vi "信号定位2.vi"() -> ()   [LabVIEW 2013]
panel:
  in  "范围":dbl
  in  "速度m/s":dbl=1.0
  out "y":dbl
  out "x":dbl
  in  "y3":dbl
  in  "x3":dbl
  in  "y2":dbl
  in  "x2":dbl
  in  "y1":dbl
  in  "x1":dbl
  in  "signal 3":dbl
  in  "signal 2":dbl
  in  "signal 1":dbl
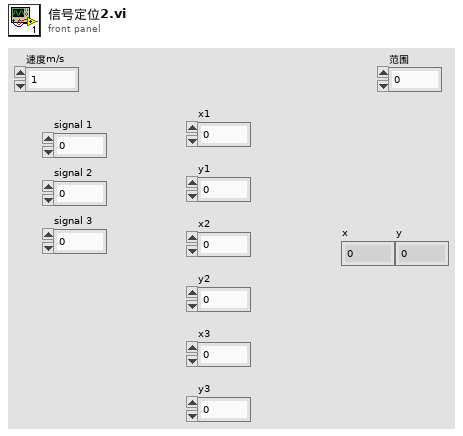
[diagram p1: front panel]
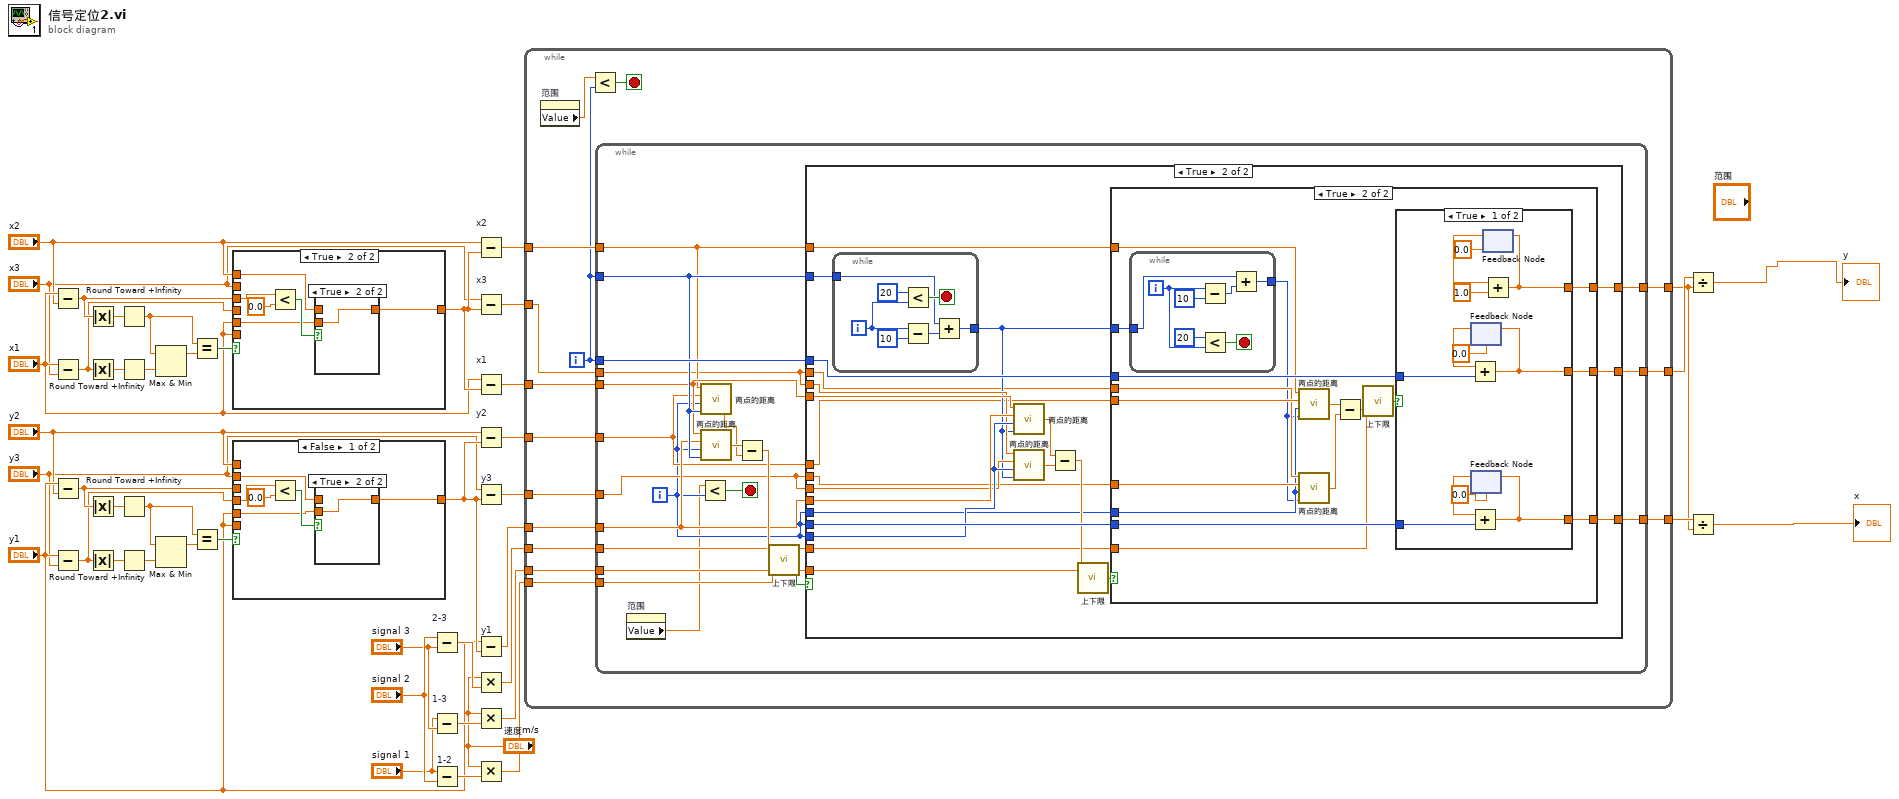
[diagram p0: block diagram]
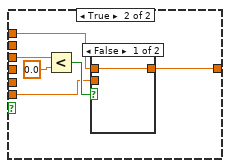
[diagram p3: hidden frame]
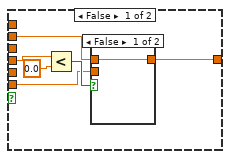
[diagram p5: hidden frame]
diagram:
  n1 = Subtract(x="x1", y="x2") -> (x-y=w24:dbl)
  n2 = Subtract(x="x1", y="x3") -> (x-y=w23:dbl)
  n3 = Subtract(x="y1", y="y2") -> (x-y=w26:dbl)
  n4 = Subtract(x="y1", y="y3") -> (x-y=w25:dbl)
  n5 = Absolute Value(x=w24) -> (abs(x)=w36:dbl)
  n6 = Absolute Value(x=w23) -> (abs(x)=w35:dbl)
  n7 = Absolute Value(x=w26) -> (abs(x)=w28:dbl)
  n8 = Absolute Value(x=w25) -> (abs(x)=w27:dbl)
  n9 = Round Toward +Infinity(x=w36) -> (ceil(x): smallest int >= x=w32:dbl)
  n10 = Round Toward +Infinity(x=w35) -> (ceil(x): smallest int >= x=w42:dbl)
  n11 = Round Toward +Infinity(x=w28) -> (ceil(x): smallest int >= x=w29:dbl)
  n12 = Round Toward +Infinity(x=w27) -> (ceil(x): smallest int >= x=w41:dbl)
  n13 = Max & Min(x=w32, y=w42) -> (max(x,y)=w33:dbl)  [unwired: 1 out]
  n14 = Max & Min(x=w29, y=w41) -> (max(x,y)=w30:dbl)  [unwired: 1 out]
  n15 = Equal?(x=w32, y=w33) -> (x = y?=w34:bool)
  n16 = Equal?(x=w29, y=w30) -> (x = y?=w31:bool)
  n17 = case shown="True" w34 {
    tunnel: w24 -> [_ w57]
    tunnel: "x1" -> [_ w56]
    tunnel: [w47 w55] -> w22
    tunnel: "x2" -> [_ w54]
    tunnel: w23 -> [w49 _]
    tunnel: "x1" -> [w48 _]
    tunnel: "x3" -> [w46 _]
    frame False {
      n18 = Less?(x=w49, y=0.0) -> (x < y?=w50:bool)
      n19 = case shown="False" w50 {
        tunnel: w48 -> [_ w53]
        tunnel: [w52 w53] -> w47
        tunnel: w46 -> [w52 _]
        frame False {
        }
        frame True {
        }
      }
    }
    frame True {
      n20 = Less?(x=w57, y=0.0) -> (x < y?=w59:bool)
      n21 = case shown="True" w59 {
        tunnel: w56 -> [_ w61]
        tunnel: [w60 w61] -> w55
        tunnel: w54 -> [w60 _]
        frame False {
        }
        frame True {
        }
      }
    }
  }
  n22 = case shown="False" w31 {
    tunnel: w26 -> [_ w73]
    tunnel: "y1" -> [_ w72]
    tunnel: [w63 w71] -> w18
    tunnel: "y2" -> [_ w70]
    tunnel: w25 -> [w65 _]
    tunnel: "y1" -> [w64 _]
    tunnel: "y3" -> [w62 _]
    frame False {
      n23 = Less?(x=w65, y=0.0) -> (x < y?=w66:bool)
      n24 = case shown="True" w66 {
        tunnel: w64 -> [_ w69]
        tunnel: [w68 w69] -> w63
        tunnel: w62 -> [w68 _]
        frame False {
        }
        frame True {
        }
      }
    }
    frame True {
      n25 = Less?(x=w73, y=0.0) -> (x < y?=w75:bool)
      n26 = case shown="False" w75 {
        tunnel: w72 -> [_ w77]
        tunnel: [w76 w77] -> w71
        tunnel: w70 -> [w76 _]
        frame False {
        }
        frame True {
        }
      }
    }
  }
  n27 = Subtract "2-3"(x="signal 2", y="signal 3") -> (x-y=w38:dbl)
  n28 = Subtract "1-3"(x="signal 1", y="signal 3") -> (x-y=w39:dbl)
  n29 = Subtract "1-2"(x="signal 1", y="signal 2") -> (x-y=w40:dbl)
  n30 = Subtract "x2"(x="x2", y=w22) -> (x-y=w12:dbl)
  n31 = Subtract "x3"(x="x3", y=w22) -> (x-y=w10:dbl)
  n32 = Subtract "x1"(x="x1", y=w22) -> (x-y=w14:dbl)
  n33 = Subtract "y2"(x="y2", y=w18) -> (x-y=w11:dbl)
  n34 = Subtract "y3"(x="y3", y=w18) -> (x-y=w9:dbl)
  n35 = Subtract "y1"(x="y1", y=w18) -> (x-y=w13:dbl)
  n36 = Multiply(x="速度m/s", y=w38) -> (x*y=w6:dbl)
  n37 = Multiply(x="速度m/s", y=w39) -> (x*y=w7:dbl)
  n38 = Multiply(x="速度m/s", y=w40) -> (x*y=w8:dbl)
  n39 = while {
    tunnel: w14 -> [w91]
    tunnel: w13 -> [w90]
    tunnel: w12 -> [w89]
    tunnel: w11 -> [w88]
    tunnel: w10 -> [w87]
    tunnel: w9 -> [w86]
    tunnel: w8 -> [w85]
    tunnel: w7 -> [w84]
    tunnel: w6 -> [w83]
    tunnel: [w81] -> w5
    tunnel: [w80] -> w4
    tunnel: [w79] -> w3
    i -> [w82]
    stop <- w92 stop-if-true
    n40 = property on="范围" class="DigNum (strict)"() -> ("Value"=w78:dbl)  [unwired: 2 in, 2 out]
    n41 = Less?(x=w78, y=w82) -> (x < y?=w92:bool)
    n42 = while {
      tunnel: w82 -> [w105]
      tunnel: w91 -> [w104]
      tunnel: w90 -> [w103]
      tunnel: w89 -> [w101]
      tunnel: w88 -> [w100]
      tunnel: w87 -> [w99]
      tunnel: w86 -> [w98]
      tunnel: w85 -> [w112]
      tunnel: w84 -> [w102]
      tunnel: w83 -> [w96]
      tunnel: w82 -> [w111]
      tunnel: [w110] -> w81
      tunnel: [w109] -> w80
      tunnel: [w108] -> w79
      i -> [w97]
      stop <- w113 stop-if-true
      n43 = property on="范围" class="DigNum (strict)"() -> ("Value"=w93:dbl)  [unwired: 2 in, 2 out]
      n44 = Less?(x=w93, y=w97) -> (x < y?=w113:bool)
      n45 = call "两点的距离.vi"("y2"=w105, "x2"=w97, "y1"=w100, "x1"=w101) -> ("de"=w94:dbl)
      n46 = call "两点的距离.vi"("y2"=w105, "x2"=w97, "y1"=w103, "x1"=w104) -> ("de"=w95:dbl)
      n47 = Subtract(x=w95, y=w94) -> (x-y=w106:dbl)
      n48 = call "上下限.vi"("要比较的"=w106, "范围的中心"=w112) -> ("T/F"=w107:bool)
      n49 = case shown="True" w107 {
        tunnel: w97 -> [_ w136]
        tunnel: w111 -> [_ w135]
        tunnel: [_ w134] -> w110
        tunnel: [_ w133] -> w109
        tunnel: [_ w132] -> w108
        tunnel: w105 -> [_ w131]
        tunnel: w97 -> [_ w130]
        tunnel: w104 -> [_ w129]
        tunnel: w103 -> [_ w128]
        tunnel: w99 -> [_ w127]
        tunnel: w98 -> [_ w126]
        tunnel: w102 -> [_ w124]
        tunnel: w101 -> [_ w121]
        tunnel: w100 -> [_ w120]
        tunnel: w99 -> [_ w119]
        tunnel: w98 -> [_ w118]
        tunnel: w97 -> [_ w117]
        tunnel: w96 -> [_ w116]
        frame False {
        }
        frame True {
          n50 = while {
            tunnel: w131 -> [w138]
            tunnel: [w137] -> w122
            i -> [w142]
            stop <- w141 stop-if-true
            n51 = Less?(x=20, y=w142) -> (x < y?=w141:bool)
            n52 = Subtract(x=w142, y=10) -> (x-y=w139:i32)
            n53 = Add(x=w138, y=w139) -> (x+y=w137:i32)
          }
          n54 = call "两点的距离.vi"("y2"=w122, "x2"=w130, "y1"=w128, "x1"=w129) -> ("de"=w115:dbl)
          n55 = call "两点的距离.vi"("y2"=w122, "x2"=w130, "y1"=w126, "x1"=w127) -> ("de"=w114:dbl)
          n56 = Subtract(x=w115, y=w114) -> (x-y=w125:dbl)
          n57 = call "上下限.vi"("要比较的"=w125, "范围的中心"=w124) -> ("T/F"=w123:bool)
          n58 = case shown="True" w123 {
            tunnel: w136 -> [_ w160]
            tunnel: w135 -> [_ w159]
            tunnel: [_ w158] -> w134
            tunnel: [_ w157] -> w133
            tunnel: [_ w156] -> w132
            tunnel: w122 -> [_ w155]
            tunnel: w121 -> [_ w153]
            tunnel: w120 -> [_ w152]
            tunnel: w119 -> [_ w151]
            tunnel: w118 -> [_ w150]
            tunnel: w117 -> [_ w149]
            tunnel: w116 -> [_ w147]
            frame False {
            }
            frame True {
              n59 = while {
                tunnel: [w162] -> w148
                tunnel: w155 -> [w161]
                i -> [w166]
                stop <- w165 stop-if-true
                n60 = Subtract(x=w166, y=10) -> (x-y=w163:i32)
                n61 = Less?(x=20, y=w166) -> (x < y?=w165:bool)
                n62 = Add(x=w161, y=w163) -> (x+y=w162:i32)
              }
              n63 = call "两点的距离.vi"("y2"=w148, "x2"=w149, "y1"=w152, "x1"=w153) -> ("de"=w145:dbl)
              n64 = call "两点的距离.vi"("y2"=w148, "x2"=w149, "y1"=w150, "x1"=w151) -> ("de"=w144:dbl)
              n65 = Subtract(x=w145, y=w144) -> (x-y=w154:dbl)
              n66 = call "上下限.vi"("要比较的"=w154, "范围的中心"=w147) -> ("T/F"=w146:bool)
              n67 = case shown="True" w146 {
                tunnel: w160 -> [w173 _]
                tunnel: w159 -> [w176 _]
                tunnel: [w172 _] -> w158
                tunnel: [w171 _] -> w157
                tunnel: [w170 _] -> w156
                frame True {
                  n68 = feedback #1(0.0) -> (w175:dbl)
                  n69 = Add(x=w175, y=w176) -> (x+y=w171:dbl)
                  n70 = feedback-in #1(w171) -> ()
                  n71 = feedback #2(0.0) -> (w174:dbl)
                  n72 = Add(x=w174, y=w173) -> (x+y=w172:dbl)
                  n73 = feedback-in #2(w172) -> ()
                  n74 = feedback #3(0.0) -> (w179:dbl)
                  n75 = Add(x=w179, y=1.0) -> (x+y=w170:dbl)
                  n76 = feedback-in #3(w170) -> ()
                }
                frame False {
                }
              }
            }
          }
        }
      }
    }
  }
  n77 = Divide(x=w4, y=w3) -> (x/y=→"y":dbl)
  n78 = Divide(x=w5, y=w3) -> (x/y=→"x":dbl)
